vi "set_autoreset.vi"(8 "error in (no error)":errorcluster, 10 "auto-reset? (T)":bool=TRUE, 11 "timer in":refnum<class "rytimer.lvclass">) -> (0 "error out":errorcluster, 3 "timer out":refnum<class "rytimer.lvclass">)   [LabVIEW 2017, in "rytimer.lvclass"]
uses:
  rytimer.lvclass
  rytimer.lvclass/rytimer.ctl
  state.ctl
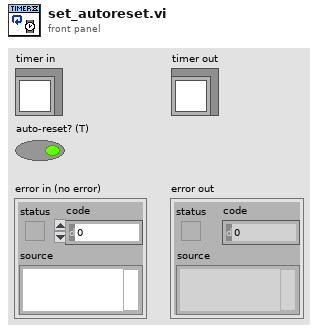
[diagram p1: front panel]
types:
  T1 = typedef "rytimer.lvclass/state.ctl" = enum8{"stop", "start", "mode", "interval", "message"}
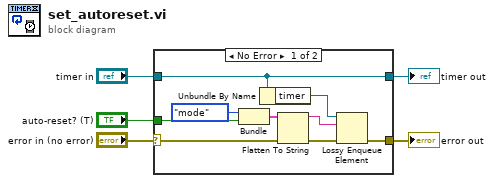
[diagram p0: block diagram]
diagram:
  n1 = case shown="No Error" "error in (no error)" {
    selector: "error in (no error)" -> [w14 w16]
    tunnel: [w13 w16] -> w4
    tunnel: "auto-reset? (T)" -> [w12 _]
    tunnel: "timer in" -> [w6 w15]
    tunnel: [w6 w15] -> w1
    frame No Error {
      n2 = Bundle("state"=state."mode", "auto-reset? (T)"=w12) -> (w7:cluster{"state":T1, "auto-reset? (T)":bool})  [unwired: 1 in]
      n3 = Unbundle By Name(w6) -> ("timer"=w11:refnum<queue>)
      n4 = Flatten To String(anything=w7, error in (no error)=w14) -> (data string=w8:string, error out=w9:errorcluster)  [unwired: 2 in, 1 out]
      n5 = Lossy Enqueue Element(queue=w11, element=w8, error in (no error)=w9) -> (error out=w13:errorcluster)  [unwired: 3 out]
    }
    frame Error {
    }
  }
  "error out" <- w4
  "timer out" <- w1
